vi "ErrorHandling.Fglb.Init.vi"(8 "error in (no error)":errorcluster) -> (0 "error out":errorcluster)   [LabVIEW 2016]
uses:
  ErrorHandling.Fglb.Action.ctl
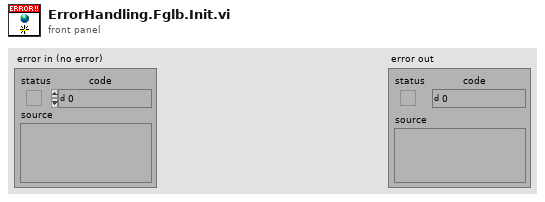
[diagram p1: front panel]
types:
  T1 = typedef "ErrorHandling.Fglb.Action.ctl" = enum16{"init", "add", "clear", "confirm", "check", "get"}
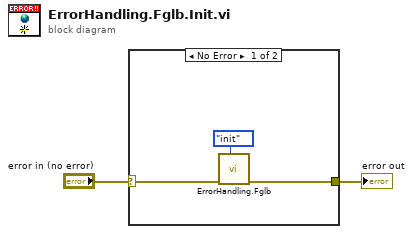
[diagram p0: block diagram]
diagram:
  n1 = case shown="No Error" "error in (no error)" {
    selector: "error in (no error)" -> [w4 w6]
    tunnel: [w5 w6] -> w2
    frame No Error {
      n2 = call "ErrorHandling.Fglb.vi"("Action"=ErrorHandling.Fglb.Action."init", "error in (no error)"=w4) -> ("error out"=w5:errorcluster)  [unwired: 7 in, 2 out]
    }
    frame Error {
    }
  }
  "error out" <- w2
